vi "Set Path.vi"(8 "error in (no error)":errorcluster, 10 "path":string, 11 "session in":T1) -> (0 "error out":errorcluster, 3 "session out":T1)   [LabVIEW 2020, in "SLSC Switch.lvlib"]
doc: "Connects two channels by specifying an explicit path in the <B>path</B> parameter. This VI is useful where path repeatability is important, such as in calibrated signal paths. If path repeatability is not necessary, use SLSC Switch.lvlib:Connect Channels.\n\nTo obtain the exact path for a given connection, use SLSC Switch.lvlib:Get Path."
uses:
  <vilib>/SLSC_Switch/SLSC Switch.lvlib
  nislscsl.dll
  <vilib>/userdefined/High Color/SLSC_Switch/nislscslSession.ctl
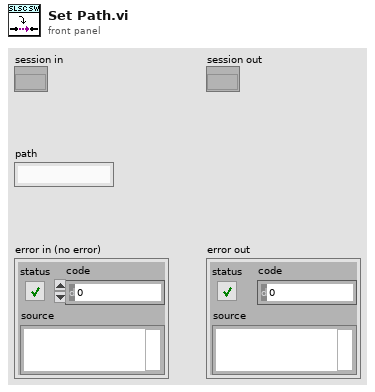
[diagram p1: front panel]
types:
  T1 = typedef "nislscslSession.ctl" = refnum<k20>
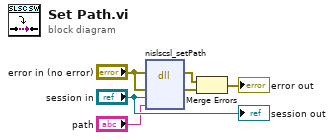
[diagram p0: block diagram]
diagram:
  n1 = dll-call lib="nislscsl.*" fn="nislscsl_setPath"(error in="error in (no error)", "errorCluster"="error in (no error)", "sessionHandle"="session in", "path"="path") -> (error out=w6:errorcluster, "errorCluster"=w5:errorcluster)  [unwired: 5 in, 1 out]
  n2 = Merge Errors(w6, w5) -> (→"error out":errorcluster)
  "session out" <- "session in"
